vi "sc5511a_set_clock_reference.vi"(0 "deviceHandle":u32 format="%.0x", 2 "Ref Output":u8(ring) items=["10 MHz", "100 MHz"], 3 "Lock external":u8(ring) items=["disable", "enable"], 5 "error in":errorcluster) -> (14 "deviceHandle":u32 format="%.0x", 19 "error out":errorcluster)   [LabVIEW 2010]
uses:
  sc5511a.dll
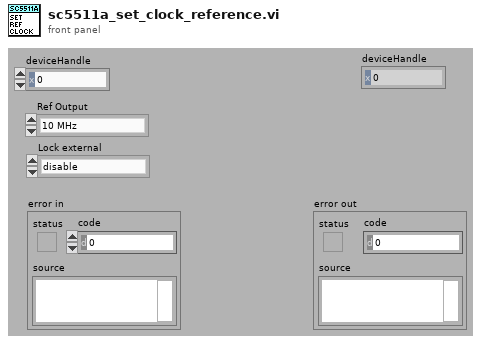
[diagram p1: front panel]
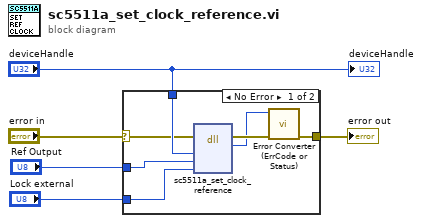
[diagram p0: block diagram]
diagram:
  n1 = case shown="No Error" "error in" {
    selector: "error in" -> [w7 w13]
    tunnel: [w12 w13] -> w5
    tunnel: "deviceHandle" -> [w9 _]
    tunnel: "Lock external" -> [w8 _]
    tunnel: "Ref Output" -> [w6 _]
    frame No Error {
      n2 = dll-call lib="sc5511a.dll" fn="sc5511a_set_clock_reference"(error in=w7, "deviceHandle"=w9, "output_high"=w6, "lock_external"=w8) -> (error out=w11:errorcluster, "return type"=w10:i32)  [unwired: 5 in, 1 out]
      n3 = call "Error Converter (ErrCode or Status).vi"("error in (no error)"=w11, "error code"=w10) -> ("error out"=w12:errorcluster)  [unwired: 9 in]
    }
    frame Error {
    }
  }
  "error out" <- w5
  "deviceHandle" <- "deviceHandle"
